vi "Read IPS Switch Heater.vi"(8 "error in (no error)":errorcluster, 11 "Instrument.Oxford1820 in":refnum<class "Instrument.Oxford1820.lvclass">) -> (0 "error out":errorcluster, 1 "Heater On?":bool, 2 "Switch Heater Status":string, 3 "Instrument.Oxford1820 out":refnum<class "Instrument.Oxford1820.lvclass">)   [LabVIEW 2019, in "Instrument.Oxford1820.lvclass"]
uses:
  Instrument.Oxford1820.lvclass
  Instrument.Oxford1820.lvclass/Instrument.Oxford1820.ctl
  <instrlib>/Mercury iXX/Public/Libraries/Magnet/Open/Open Magnet Device.vi
  <instrlib>/Mercury iXX/Public/Libraries/Magnet/Signals/Read/Switch Heater Status (Read).vi
  <instrlib>/Mercury iXX/Mercury iXX.lvlib
  <instrlib>/Mercury iXX/Public/Libraries/Magnet.lvlib
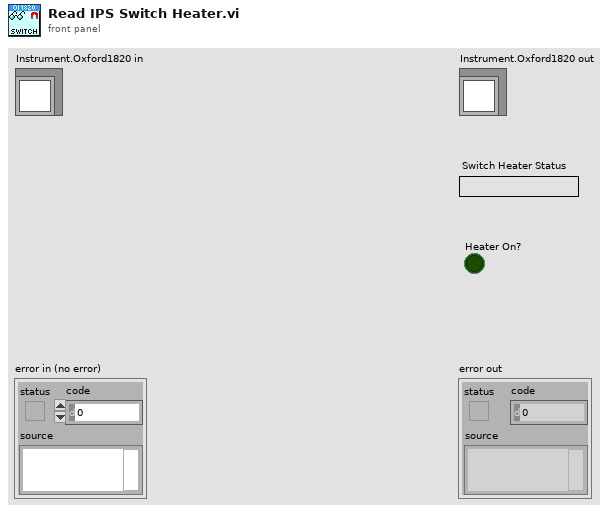
[diagram p1: front panel]
types:
  T1 = typedef "Mercury iXX.lvlib/Mercury Reference.ctl" = cluster{"Comms":refnum<visa-resource-name>, "Device ID":string[], "Comms Layer":T2, "Command":string, "Query reference":T3}
  T2 = typedef "Mercury iXX.lvlib/Comms Transport Layer.ctl" = enum16{"Ethernet TCP/IP", "USB", "ISOBus - RS-232", "GPIB"}
  T3 = typedef "Mercury iXX.lvlib/Query Dynamic Reference.ctl" = refnum<vi>
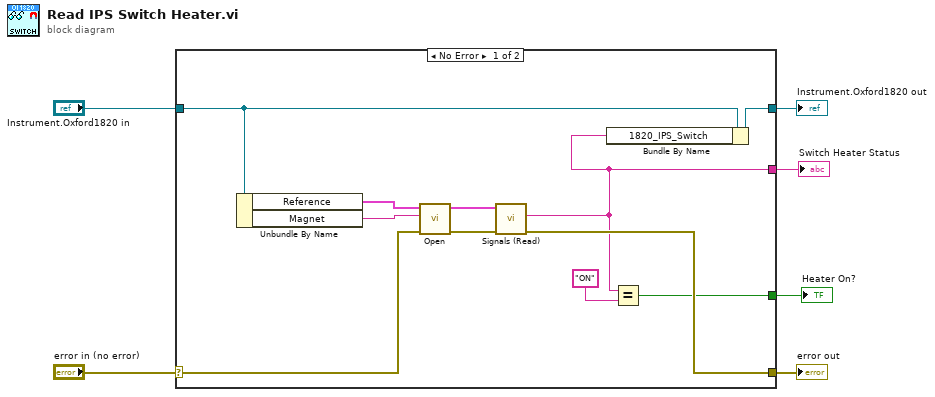
[diagram p0: block diagram]
diagram:
  n1 = case shown="No Error" "error in (no error)" {
    selector: "error in (no error)" -> [w13 w19]
    tunnel: [w12 w19] -> w5
    tunnel: [w8 w18] -> w3
    tunnel: "Instrument.Oxford1820 in" -> [w7 w18]
    tunnel: [w9 _] -> w2
    tunnel: [w10 _] -> w1
    frame No Error {
      n2 = Unbundle By Name(w7) -> ("Reference"=w14:T1, "Magnet"=w15:string)
      n3 = call-poly <instrlib>:"Open.vi"("error in (no error)"=w13, "Device Identifier"=w15, "Mercury Reference In"=w14) -> ("error out"=w17:errorcluster, "Mercury Reference Out"=w16:T1)  [unwired: 7 out]
      n4 = call-poly <instrlib>:"Signals (Read).vi"("error in"=w17, "Mercury Reference In"=w16) -> ("error out"=w12:errorcluster, "Switch Heater Status"=w9:string)  [unwired: 1 in, 7 out]
      n5 = Bundle By Name(cluster=w7, "1820_IPS_Switch"=w9) -> (w8:refnum<class "Instrument.Oxford1820.lvclass">)
      n6 = Equal?(x=w9, y="ON") -> (x = y?=w10:bool)
    }
    frame Error {
    }
  }
  "error out" <- w5
  "Instrument.Oxford1820 out" <- w3
  "Switch Heater Status" <- w2
  "Heater On?" <- w1
